vi "Get Size.vi"(8 "error in (no error)":errorcluster, 11 "Picture Control Canvas in":refnum<class "Tree Control Canvas.lvclass">) -> (0 "error out":errorcluster, 2 "Size":cluster{"Width":u16, "Height":u16}, 3 "Picture Control Canvas out":refnum<class "Tree Control Canvas.lvclass">)   [LabVIEW 2023, in "Font Glyph Drawer Interface.lvlib" / "Tree Control Canvas.lvclass"]
uses:
  Tree Control Canvas.lvclass
  Tree Control Canvas.lvclass/Tree Control Canvas.ctl
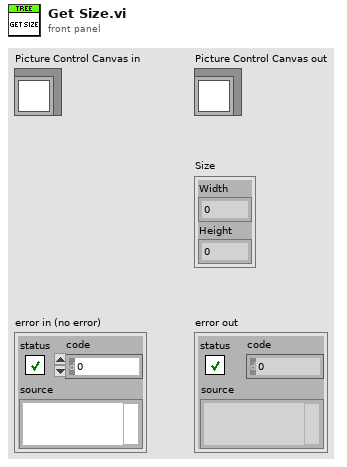
[diagram p1: front panel]
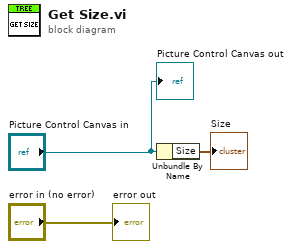
[diagram p0: block diagram]
diagram:
  n1 = Unbundle By Name("Picture Control Canvas in") -> ("Size"=→"Size":cluster{"Width":u16, "Height":u16})
  "error out" <- "error in (no error)"
  "Picture Control Canvas out" <- "Picture Control Canvas in"
